vi "6-2 hp34401 idn.vi"(0 "adr":string="4") -> (1 "error out":errorcluster, 2 "data sel (anno)":string, 3 "data":string, 4 "idn":string)   [LabVIEW 2012]
panel:
  # "2. TEST INVIO RICHIESTE E RICEZIONE RISPOSTE dallo STRUMENTO\n    Realizzare un VI che interroghi lo strumento per ottenere la sua identificazione (comando *IDN?) \n    e l'anno della versione  del linguaggio SCPI supportata (syst:vers?)."
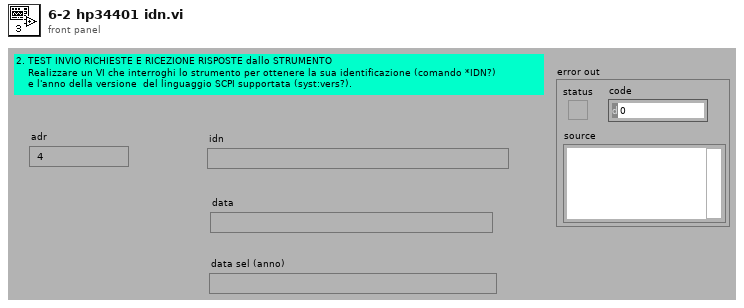
[diagram p1: front panel]
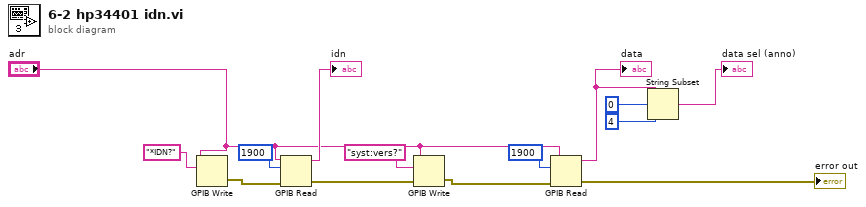
[diagram p0: block diagram]
diagram:
  n1 = GPIB Write(0:"adr", 1:"*IDN?" ("data")) -> (6:w8:errorcluster)  [unwired: 3 in, 1 out]
  n2 = GPIB Read(0:"adr", 1:1900 ("timeout ms (488.2 global)"), 3:w8) -> (5:→"idn":string, 7:w7:errorcluster)  [unwired: 2 in, 1 out]
  n3 = GPIB Write(0:"adr", 1:"syst:vers?" ("data"), 3:w7) -> (6:w12:errorcluster)  [unwired: 2 in, 1 out]
  n4 = GPIB Read(0:"adr", 1:1900 ("timeout ms (488.2 global)"), 3:w12) -> (5:w5:string, 7:→"error out":errorcluster)  [unwired: 2 in, 1 out]
  "data" <- w5
  n5 = String Subset(string=w5, offset (0)=0, length (rest)=4 ("length (rest)")) -> (substring=→"data sel (anno)":string)
